vi "Summary.vi"(8 "error in":errorcluster, 10 "depth":i32, 11 "node self ref":refnum<data-value>) -> (0 "error out":errorcluster, 2 "summary":T1[](array[typedef]))   [LabVIEW 2025, in "CEF.lvlib"]
doc: "Gets the summary of a node and all the subnodes. This description can be used to update the tree controlCopyright 2017 National Instruments Corporation\n\nLicensed under the Apache License, Version 2.0 (the \"License\"); you may not use this file except in compliance with the License. You may obtain a copy of the License at http://www.apache.org/licenses/LICENSE-2.0\nUnless required by applicable law or agreed to in writing, software distributed under the License is distributed on an \"AS IS\" BASIS, WITHOUT WARRANTIES OR CONDITIONS OF ANY KIND, either express or implied. See the License for the specific language governing permissions and limitations under the License."
uses:
  CEF.lvlib
  Node/Summary.ctl
  Node/CEF_Node.lvclass
  Node/CEF_Node.lvclass/CEF_Node.ctl
  Node/ReadParent.vi
  Node/ReadChildren.vi
  Node/ReadNodeClass.vi
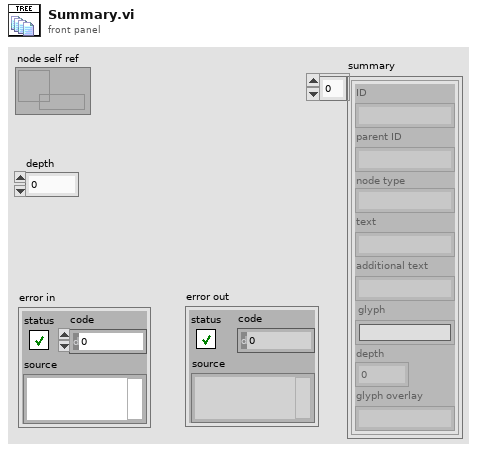
[diagram p1: front panel]
types:
  T1 = typedef "CEF.lvlib/CEF_Node.lvclass/Summary.ctl" = cluster{"ID":string, "parent ID":string, "node type":string, "text":string, "additional text":string, "glyph":string, "depth":i32, "glyph overlay":string}
  T2 = typedef "CEF.lvlib/CEF_Node.lvclass/NodeRef.ctl" = refnum<data-value>
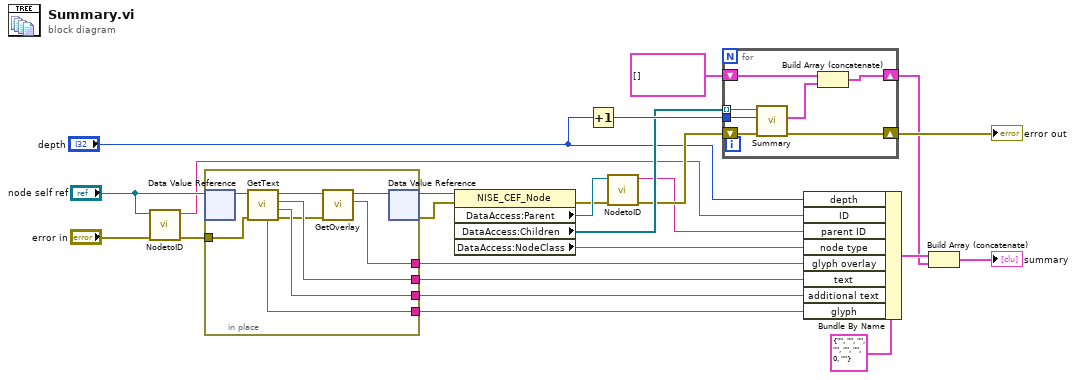
[diagram p0: block diagram]
diagram:
  n1 = call "NodetoID.vi"("error in"="error in", "node ref"="node self ref") -> ("error out"=w11:errorcluster, "ID"=w2:string)  [unwired: 8 in]
  n2 = in-place {
    in-place-border: [w33] -> w19
    in-place-border: [w32] -> w6
    in-place-border: [w31] -> w18
    in-place-border: w11 -> [w30]
    in-place-border: [w25] -> w5
    n3 = in-place-dvr #1("node self ref") -> (w29:refnum<class "CEF_Node.lvclass">)  [unwired: 1 out]
    n4 = call-dynamic "GetText.vi"("error in"=w30, "CEF_Node in"=w29) -> ("error out"=w26:errorcluster, "additional text"=w33:string, "text"=w32:string, "CEF_Node out"=w28:refnum<class "CEF_Node.lvclass">, "glyph"=w31:string)  [unwired: 5 in]
    n5 = call-dynamic "GetOverlay.vi"("error in"=w26, "CEF_Node in"=w28) -> ("overlay"=w25:string, "CEF_Node out"=w27:refnum<class "CEF_Node.lvclass">)  [unwired: 7 in, 1 out]
    n6 = in-place-dvr #1(w27) -> (w10:refnum<data-value>, w9:errorcluster)
  }
  n7 = property class="NISE_CEF_Node"(reference=w10, error in=w9) -> (error out=w8:errorcluster, "DataAccess:Parent"=w12:T2, "DataAccess:Children"=w13:T2[], "DataAccess:NodeClass"=w4:string)  [unwired: 1 out]
  n8 = Increment(x="depth") -> (x+1=w17:i32)
  n9 = call "NodetoID.vi"("error in"=w8, "node ref"=w12) -> ("error out"=w7:errorcluster, "ID"=w1:string)  [unwired: 8 in]
  n10 = for {
    tunnel: w13 -> [w36] mode=indexing
    tunnel: w17 -> [w40]
    shift-right: [w38] -> w14
    shift-left: T1[] [] ("childrensummary") -> [w39]
    shift-right: [w34] -> w23
    shift-left: w7 -> [w35]
    n11 = call "Summary.vi"("error in"=w35, "depth"=w40, "node self ref"=w36) -> ("error out"=w34:errorcluster, "summary"=w37:T1[])  [unwired: 7 in]
    n12 = Build Array (concatenate)(w39, w37) -> (w38:T1[])
  }
  "error out" <- w23
  n13 = Bundle By Name(cluster=T1 {"ID"="", "parent ID"="", "node type"="", "text"="", "additional text"="", "glyph"="", "depth"=0, "glyph overlay"=""} ("nodeSummary"), "depth"="depth", "ID"=w2, "parent ID"=w1, "node type"=w4, "glyph overlay"=w5, "text"=w6, "additional text"=w19, "glyph"=w18) -> (w15:T1)
  n14 = Build Array (concatenate)(w15, w14) -> (→"summary":T1[])
